vi "taskPrototype.vi"(8 "error in (no error)":errorcluster, 10 "taskChannel":refnum<class "ITaskChannel.lvclass">, 11 "ITask in":refnum<class "ITask.lvclass">) -> (0 "error out":errorcluster, 3 "ITask out":refnum<class "ITask.lvclass">)   [LabVIEW 2023]
uses:
  ITask/ITask.lvclass
  ITaskChannel/ITaskChannel.lvclass
  BoolNotifierTaskChannel/BoolNotifierTaskChannel.lvclass
  Examples/Example_Bool_Notifier_StopMech/Task_BoolStopNotifier/Task_BoolStopNotifier.lvclass
  BoolNotifierTaskChannel/BoolNotifierTaskChannel.lvclass/BoolNotifierTaskChannel.ctl
  BoolNotifierTaskChannel/Read notifierRef.vi
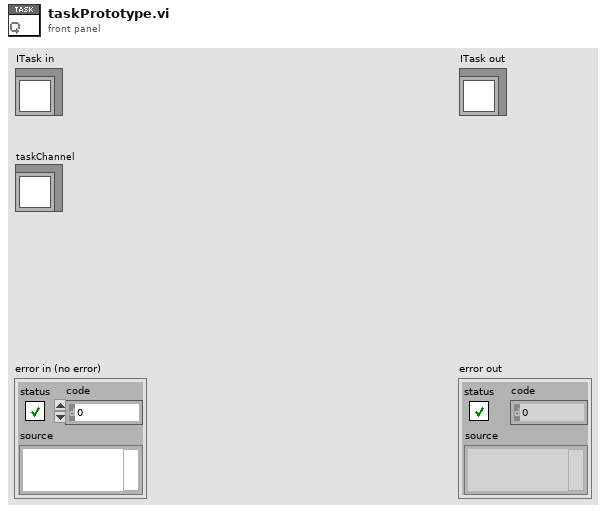
[diagram p1: front panel]
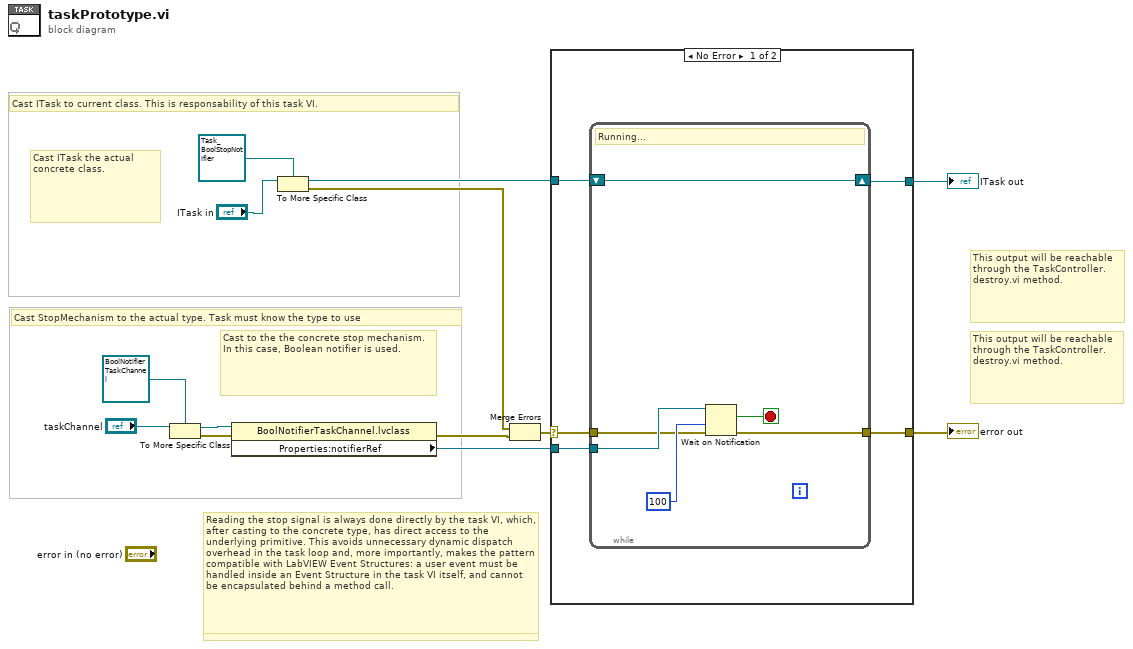
[diagram p0: block diagram]
diagram:
  # "This output will be reachable through the TaskController.destroy.vi method."
  # "This output will be reachable through the TaskController.destroy.vi method."
  # "Cast ITask the actual concrete class."
  # "Reading the stop signal is always done directly by the task VI, which, after casting to the concrete type, has direct access to the underlying primitive. This avoids unnecessary dynamic dispatch overhead in the task loop and, more importantly, makes the pattern compatible with LabVIEW Event Structures: a user event must be handled inside an Event Structure in the task VI itself, and cannot be encapsulated behind a method call."
  # "Cast to the the concrete stop mechanism.\nIn this case, Boolean notifier is used."
  # "Reading the stop signal is always done directly by the task VI, which, after casting to the concrete type, has direct access to the underlying primitive. This avoids unnecessary dynamic dispatch overhead in the task loop and, more importantly, makes the pattern compatible with LabVIEW Event Structures: a user event must be handled inside an Event Structure in the task VI itself, and cannot be encapsulated behind a method call."
  # "Cast ITask to current class. This is responsability of this task VI."
  # "Cast StopMechanism to the actual type. Task must know the type to use"
  n1 = To More Specific Class(target class=refnum<class "BoolNotifierTaskChannel.lvclass"> refnum ("TLC_Daemon.lvlib:NotifierStopMechanism.lvclass"), reference="taskChannel") -> (specific class reference=w10:refnum<class "BoolNotifierTaskChannel.lvclass">, error out=w7:errorcluster)  [unwired: 1 in]
  n2 = property class="BoolNotifierTaskChannel.lvclass"(reference=w10, error in=w7) -> (error out=w6:errorcluster, "Properties:notifierRef"=w9:refnum<notifier>)  [unwired: 1 out]
  n3 = To More Specific Class(target class=refnum<class "Task_BoolStopNotifier.lvclass"> refnum ("ExampleTask_StopNotifier.lvclass"), reference="ITask in") -> (specific class reference=w8:refnum<class "Task_BoolStopNotifier.lvclass">, error out=w11:errorcluster)  [unwired: 1 in]
  n4 = Merge Errors(w11, w6) -> (w5:errorcluster)
  n5 = case shown="No Error" w5 {
    selector: w5 -> [w17 w26]
    tunnel: w9 -> [w18 _]
    tunnel: w8 -> [w15 w25]
    tunnel: [w14 w25] -> w1
    tunnel: [w16 w26] -> w2
    frame No Error {
      n6 = while {
        tunnel: w18 -> [w24]
        tunnel: w17 -> [w21]
        tunnel: [w20] -> w16
        shift-right: [w19] -> w14
        shift-left: w15 -> [w19]
        stop <- w22 stop-if-true
        # "Running..."
        n7 = Wait on Notification(notifier=w24, timeout in ms (-1)=100, error in (no error)=w21) -> (notification=w22:bool, error out=w20:errorcluster)  [unwired: 1 in, 2 out]
      }
    }
    frame Error {
    }
  }
  "error out" <- w2
  "ITask out" <- w1
